vi "Read All Stderr.vi"(6 "Per Read Size":i32=1024 max=30000, 8 "Error In":errorcluster, 10 "Total Read Size":i32=1024, 11 "Channel In":refnum<class "Channel.lvclass">) -> (0 "Error Out":errorcluster, 1 "Timed Out?":bool, 2 "Data":u8[](array[numeric]), 3 "Channel Out":refnum<class "Channel.lvclass">)   [LabVIEW 2021, in "Field_RnD_Services_LIBSSH2_Toolkit.lvlib" / "Channel.lvclass"]
doc: "Reads binary data from the STDERR stream of a SSH channel represented by this Channel object in chunks, or blocks, until the total read size is reached. This VI should be used if the <B>Total Read Size</B> is greater than 30KB because of a hard-coded per-read maximum of 30KB defined in the libssh2 shared library."
uses:
  Channel.lvclass
  Channel.lvclass/Channel.ctl
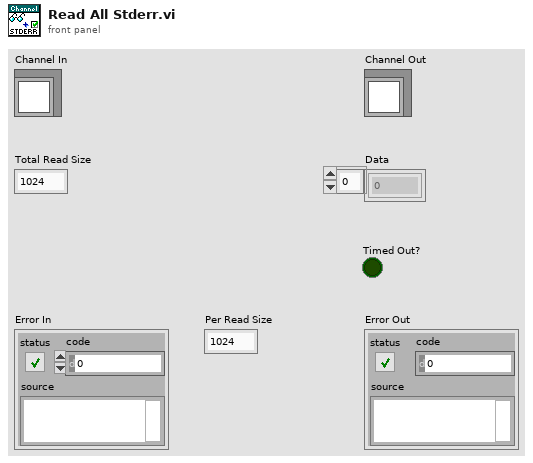
[diagram p1: front panel]
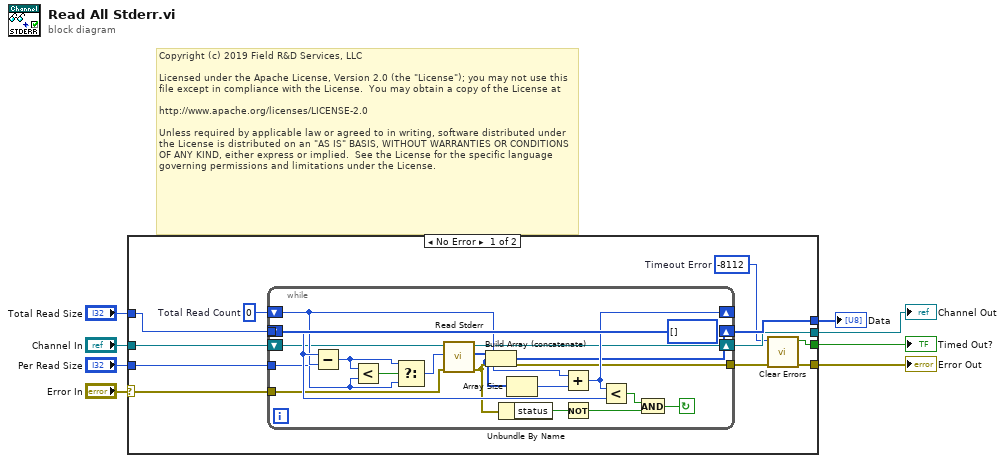
[diagram p0: block diagram]
diagram:
  # "Copyright (c) 2019 Field R&D Services, LLC\n\nLicensed under the Apache License, Version 2.0 (the \"License\"); you may not use this file except in compliance with the License.  You may obtain a copy of the License at\n\nhttp://www.apache.org/licenses/LICENSE-2.0\n\nUnless required by applicable law or agreed to in writing, software distributed under the License is distributed on an \"AS IS\" BASIS, WITHOUT WARRANTIES OR CONDITIONS OF ANY KIND, either express or implied.  See the License for the specific language governing permissions and limitations under the License."
  n1 = case shown="No Error" "Error In" {
    selector: "Error In" -> [w14 w40]
    tunnel: "Total Read Size" -> [w19 _]
    tunnel: "Per Read Size" -> [w18 _]
    tunnel: "Channel In" -> [w17 w41]
    tunnel: [w16 _] -> w5
    tunnel: [w15 w41] -> w4
    tunnel: [w12 w40] -> w3
    tunnel: [w10 _] -> w1
    frame No Error {
      w11 = -8112  # Timeout Error
      w20 = 0  # Total Read Count
      n2 = while {
        shift-right: [w32] -> w15
        shift-left: w17 -> [w29]
        shift-right: [w38] -> _
        shift-left: w20 -> [w36]
        tunnel: w19 -> [w37]
        tunnel: w18 -> [w33]
        tunnel: w14 -> [w28]
        tunnel: [w25] -> w13
        shift-right: [w21] -> w16
        shift-left: u8[] [] ("Data") -> [w22]
        stop <- w23 continue-if-true
        n3 = Subtract(x=w37, y=w36) -> (x-y=w34:i32)
        n4 = Less?(x=w34, y=w33) -> (x < y?=w35:bool)
        n5 = Select(t=w34, s=w35, f=w33) -> (s? t:f=w30:i32)
        n6 = call "Read Stderr.vi"("Error In"=w28, "Max Data Length"=w30, "Channel In"=w29) -> ("Error Out"=w25:errorcluster, "Data"=w31:u8[], "Channel Out"=w32:refnum<class "Channel.lvclass">)  [unwired: 6 in]
        n7 = Build Array (concatenate)(w22, w31) -> (w21:u8[])
        n8 = Unbundle By Name(w25) -> ("status"=w24:bool)
        n9 = Array Size(array=w31) -> (size(s)=w39:i32)
        n10 = Add(x=w36, y=w39) -> (x+y=w38:i32)
        n11 = Not(x=w24) -> (.not. x?=w27:bool)
        n12 = Less?(x=w38, y=w37) -> (x < y?=w26:bool)
        n13 = And(x=w26, y=w27) -> (x .and. y?=w23:bool)
      }
      n14 = call <vilib>:"Clear Errors.vi"("error in (no error)"=w13, "specific error code to clear (0: all)"=w11) -> ("error out"=w12:errorcluster, "specific error cleared?"=w10:bool)  [unwired: 4 in]
    }
    frame Error {
    }
  }
  "Data" <- w5
  "Channel Out" <- w4
  "Error Out" <- w3
  "Timed Out?" <- w1
